vi "Get Sheet byName.vi"(8 "error IO":errorcluster, 10 "SheetName":string, 11 "ooCalc in":refnum<class "ooCalc.lvclass">) -> (0 "error out":errorcluster, 2 "Sheet":refnum<k24>, 3 "ooCalc out":refnum<class "ooCalc.lvclass">)   [LabVIEW 2009, in "ooCalc.lvclass"]
uses:
  ooCalc.lvclass
  C:/Projets/LAVAG/OpenOfficeRGT/AODL/DLLs/AODL.dll
  ooCalc.lvclass/ooCalc.ctl
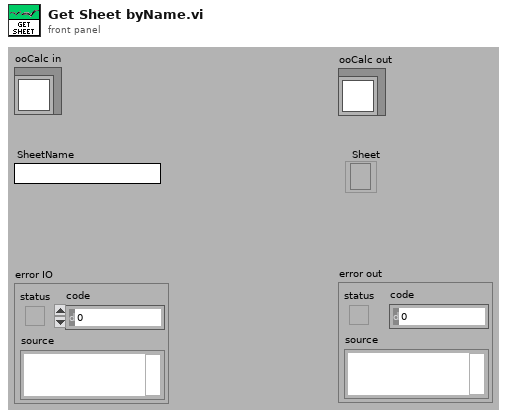
[diagram p1: front panel]
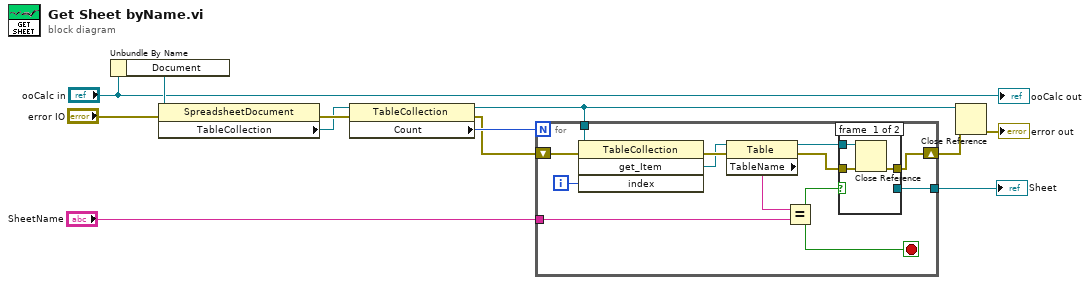
[diagram p0: block diagram]
diagram:
  n1 = Unbundle By Name("ooCalc in") -> ("Document"=w9:refnum<k24>)
  n2 = property class="SpreadsheetDocument"(reference=w9, error in="error IO") -> (error out=w11:errorcluster, "TableCollection"=w7:refnum<k24>)  [unwired: 1 out]
  n3 = property class="TableCollection"(reference=w7, error in=w11) -> (reference out=w5:refnum<k24>, error out=w4:errorcluster, "Count"=w6:i32)
  n4 = for {
    N: w6 -> [_]
    tunnel: w5 -> [w21]
    shift-right: [w19] -> w3
    shift-left: w4 -> [w20]
    tunnel: "SheetName" -> [w16]
    tunnel: [w14] -> w1
    i -> [w24]
    stop <- w13 stop-if-true
    n5 = invoke class="TableCollection" method="get_Item"(reference=w21, error in=w20, "index"=w24) -> (error out=w23:errorcluster, "get_Item"=w17:refnum<k24>)  [unwired: 1 in, 2 out]
    n6 = property class="Table"(reference=w17, error in=w23) -> (reference out=w22:refnum<k24>, error out=w18:errorcluster, "TableName"=w15:string)
    n7 = Equal?(x=w15, y=w16) -> (x = y?=w13:bool)
    n8 = case shown="False" w13 {
      tunnel: w22 -> [w27 w29]
      tunnel: [w26 w28] -> w19
      tunnel: w18 -> [w25 w28]
      tunnel: [_ w29] -> w14
      frame #0 {
        n9 = Close Reference(reference=w27, error in (no error)=w25) -> (error out=w26:errorcluster)
      }
      frame #1 {
      }
    }
  }
  "Sheet" <- w1
  n10 = Close Reference(reference=w5, error in (no error)=w3) -> (error out=→"error out":errorcluster)
  "ooCalc out" <- "ooCalc in"
